vi "PrepareSignals.vi"(6 "ListOfBases_Data":refnum<vi>, 7 "SetValueInfo in":refnum<vi>[](array[refnum]), 8 "setfile path":path, 9 "Enum":enum16{"Save", "Load"}(ring), 10 "Display Message to \nUser":bool=TRUE, 11 "DIMControSet in":refnum<vi>[](array[refnum])) -> (0 "indexed loaded Array":dbl[][](array[numeric]), 1 "Name Array":string[](array[string]), 3 "DIMControSet out":refnum<vi>[](array[refnum]))   [LabVIEW 2014, in "Panels.lvlib"]
uses:
  Panels.lvlib
  Instance           1 22Saved   PrepareSignals .vi
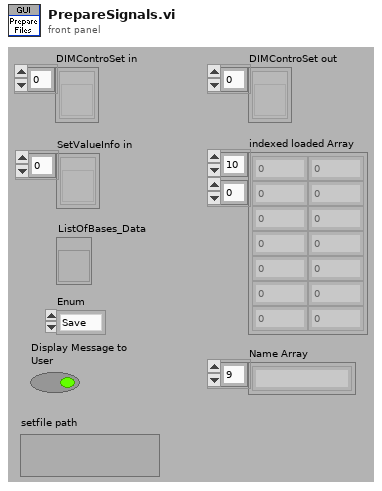
[diagram p1: front panel]
types:
  T1 = enum16{"open", "replace", "create", "open or create", "replace or create", "replace or create with confirmation"}
  T2 = cluster{"data":dbl[], "no link":bool, "quality":i32, "timeStamp":dbl}
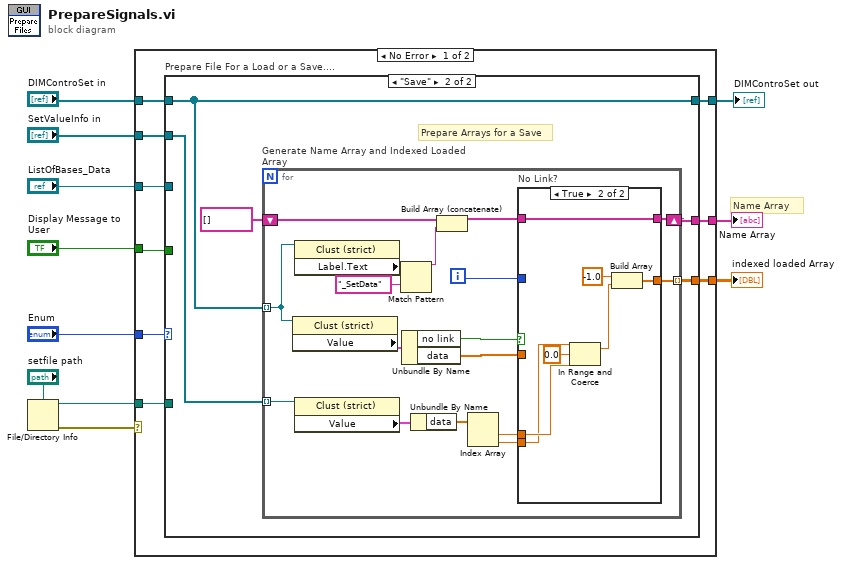
[diagram p0: block diagram]
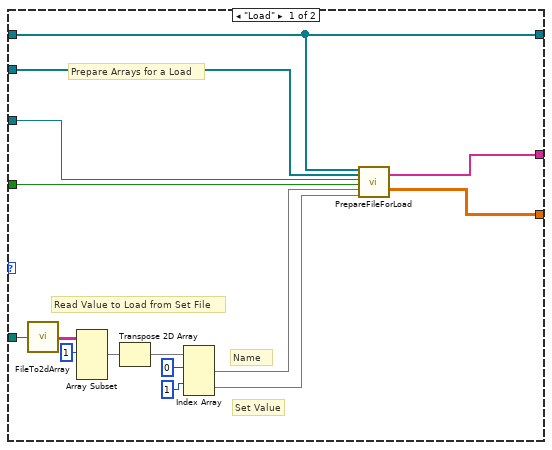
[diagram p2: hidden frame]
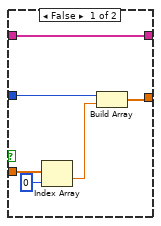
[diagram p3: hidden frame]
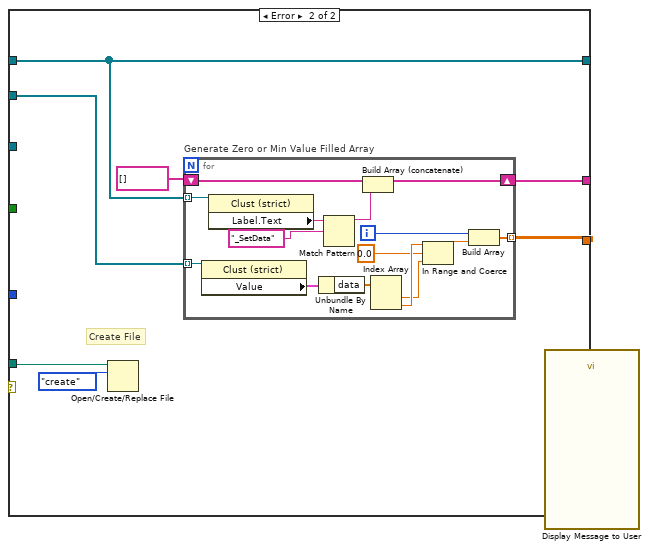
[diagram p4: hidden frame]
diagram:
  # "Name Array"
  n1 = File/Directory Info(path="setfile path") -> (path out=w7:path, error out=w11:errorcluster)  [unwired: 1 in, 5 out]
  n2 = case shown="No Error" w11 {
    tunnel: w7 -> [w18 w72]
    tunnel: "DIMControSet in" -> [w20 w77]
    tunnel: [w13 w76] -> w10
    tunnel: [w17 w77] -> w5
    tunnel: [w19 w74] -> w9
    tunnel: "Enum" -> [w16 _]
    tunnel: "Display Message to \nUser" -> [w15 _]
    tunnel: "SetValueInfo in" -> [w14 w71]
    tunnel: "ListOfBases_Data" -> [w12 _]
    frame No Error {
      n3 = case "Prepare File For a Load or a Save...." shown="\"Save\"" w16 {
        tunnel: w20 -> [w28 w38]
        tunnel: [w24 w39] -> w19
        tunnel: w18 -> [w29 _]
        tunnel: [w28 w38] -> w17
        tunnel: w15 -> [w27 _]
        tunnel: w14 -> [w22 w37]
        tunnel: [w23 w36] -> w13
        tunnel: w12 -> [w21 _]
        frame "Load" {
          # "Set Value"
          # "Name"
          # "Read Value to Load from Set File"
          # "Prepare Arrays for a Load"
          n4 = call "FileTo2dArray.vi"("file path (dialog if empty)"=w29) -> ("Array"=w35:string[][])
          n5 = Array Subset(array=w35, index (row)=1 ("index")) -> (w30:string[][])  [unwired: 3 in]
          n6 = Transpose 2D Array(2D array=w30) -> (transposed array=w31:string[][])
          n7 = Index Array(array=w31, index (row) #1=0 ("index"), index (row) #2=1 ("index")) -> (element #1=w26:string[], element #2=w25:string[])  [unwired: 2 in]
          n8 = call "PrepareFileForLoad.vi"("DIMControSet in"=w28, "SetValueInfo in"=w22, "ListOfBases_Data"=w21, "Display Message"=w27, "Load Value Name Array"=w26, "Load Value Array"=w25) -> ("Name Array"=w24:string[], "indexed loaded Array"=w23:dbl[][])  [unwired: 12 in]
        }
        frame "Save" {
          # "Prepare Arrays for a Save"
          n9 = for "Generate Name Array and Indexed Loaded Array" {
            tunnel: [w57] -> w36 mode=indexing
            tunnel: w38 -> [w55] mode=indexing
            shift-right: [w52] -> w39
            shift-left: string[] [] ("array") -> [w50]
            tunnel: w37 -> [w45] mode=indexing
            i -> [w51]
            n10 = property class="Clust (strict)"(reference=w55) -> ("Value"=w47:T2)  [unwired: 1 in, 2 out]
            n11 = property class="Clust (strict)"(reference=w55) -> ("Label.Text"=w53:string)  [unwired: 1 in, 2 out]
            n12 = property class="Clust (strict)"(reference=w45) -> ("Value"=w44:T2)  [unwired: 1 in, 2 out]
            n13 = Match Pattern(string=w53, regular expression="_SetData") -> (before substring=w48:string)  [unwired: 1 in, 3 out]
            n14 = Unbundle By Name(w47) -> ("no link"=w56:bool, "data"=w46:dbl[])
            n15 = Unbundle By Name(w44) -> ("data"=w43:dbl[])
            n16 = Build Array (concatenate)(w50, w48) -> (w49:string[])
            n17 = Index Array(array=w43) -> (element #1=w42:dbl, element #2=w41:dbl)  [unwired: 2 in]
            n18 = case "No Link?" shown="True" w56 {
              tunnel: w46 -> [w62 _]
              tunnel: [w63 w64] -> w57
              tunnel: [w60 w70] -> w52
              tunnel: w49 -> [w60 w70]
              tunnel: w51 -> [w59 _]
              tunnel: w42 -> [_ w69]
              tunnel: w41 -> [_ w68]
              frame False {
                n19 = Index Array(array=w62, index=0) -> (element=w61:dbl)
                n20 = Build Array(w59, w61) -> (w63:dbl[])
              }
              frame True {
                n21 = In Range and Coerce(upper limit=w68, x=0.0, lower limit=w69) -> (coerced(x)=w65:dbl)  [unwired: 1 out]
                n22 = Build Array(-1.0 ("element"), w65) -> (w64:dbl[])
              }
            }
          }
        }
      }
    }
    frame Error {
      # "Create File"
      n23 = Open/Create/Replace File(file path (use dialog)=w72, operation (0:open)=T1."create") -> ()  [unwired: 4 in, 3 out]
      n24 = for "Generate Zero or Min Value Filled Array" {
        tunnel: w77 -> [w90] mode=indexing
        tunnel: [w88] -> w76 mode=indexing
        shift-right: [w87] -> w74
        shift-left: string[] [] ("array") -> [w86]
        tunnel: w71 -> [w84] mode=indexing
        i -> [w89]
        n25 = property class="Clust (strict)"(reference=w84) -> ("Value"=w82:T2)  [unwired: 1 in, 2 out]
        n26 = property class="Clust (strict)"(reference=w90) -> ("Label.Text"=w91:string)  [unwired: 1 in, 2 out]
        n27 = Unbundle By Name(w82) -> ("data"=w83:dbl[])
        n28 = Match Pattern(string=w91, regular expression="_SetData") -> (before substring=w85:string)  [unwired: 1 in, 3 out]
        n29 = Build Array (concatenate)(w86, w85) -> (w87:string[])
        n30 = Index Array(array=w83) -> (element #1=w80:dbl, element #2=w81:dbl)  [unwired: 2 in]
        n31 = In Range and Coerce(upper limit=w81, x=0.0 ("element"), lower limit=w80) -> (coerced(x)=w78:dbl)  [unwired: 1 out]
        n32 = Build Array(w89, w78) -> (w88:dbl[])
      }
      n33 = call "Display Message to User"() -> ()  [unwired: 10 in, 2 out]
    }
  }
  "indexed loaded Array" <- w10
  "Name Array" <- w9
  "DIMControSet out" <- w5
